vi "Get joint offsets.vi"(11 "Analytical Serial Arm Class in":refnum<class "NI_Robotics_Analytical Serial Arm Class.lvclass">) -> (2 "joint offsets":dbl[](array[numeric]), 3 "Analytical Serial Arm Class out":refnum<class "NI_Robotics_Analytical Serial Arm Class.lvclass">)   [LabVIEW 2017, in "NI_Robotics_Analytical Serial Arm Class.lvclass"]
uses:
  <vilib>/robotics/Kinematics/Analytical/Generic/NI_Robotics_Analytical Serial Arm Class.lvclass
  c:/Program Files (x86)/National Instruments/LabVIEW 2017/vi.lib/robotics/Kinematics/Robot/NI_Robotics_Serial Robot Arm.lvclass
  <vilib>/robotics/Kinematics/Link/NI_Robotics_Link.lvclass/NI_Robotics_Link.ctl
  <vilib>/robotics/Kinematics/Robot/NI_Robotics_Serial Robot Arm.lvclass
  <vilib>/robotics/Kinematics/Link/NI_Robotics_Link.lvclass
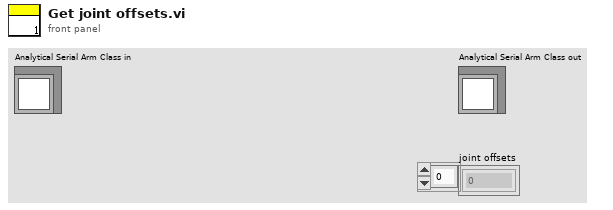
[diagram p1: front panel]
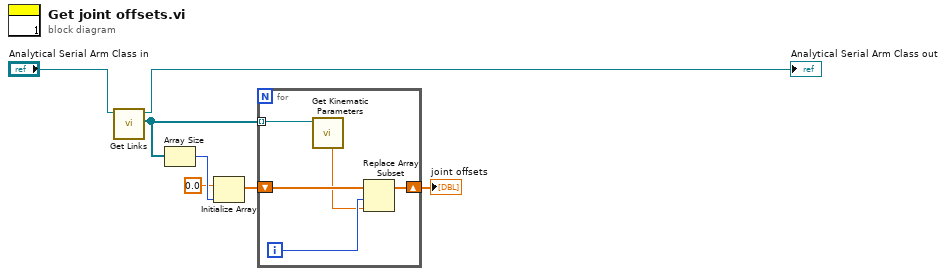
[diagram p0: block diagram]
diagram:
  n1 = call <vilib>:"Get Links.vi"("serial arm in"="Analytical Serial Arm Class in") -> ("links"=w3:refnum<class "NI_Robotics_Link.lvclass">[], "serial arm out"=→"Analytical Serial Arm Class out":refnum<class "NI_Robotics_Analytical Serial Arm Class.lvclass">)  [unwired: 8 in, 1 out]
  n2 = Array Size(array=w3) -> (size(s)=w5:i32)
  n3 = Initialize Array(0.0 ("element"), w5) -> (w2:dbl[])
  n4 = for {
    tunnel: w3 -> [w12] mode=indexing
    shift-right: [w8] -> w1
    shift-left: w2 -> [w11]
    i -> [w10]
    n5 = call <vilib>:"Get Kinematic Parameters.vi"("NI_Robotics_Link in"=w12) -> ("Joint Coordinate Offset"=w9:dbl)  [unwired: 6 in, 4 out]
    n6 = Replace Array Subset(array=w11, new element=w9, index=w10) -> (w8:dbl[])
  }
  "joint offsets" <- w1
